vi "Begin.vi"(8 "error in":errorcluster) -> (0 "error out":errorcluster)   [LabVIEW 2015]
doc: "Called before other user functions, this VI is expected to open initial I/O refnums, load in file data, and do all program initialization. Notice that the <B>error out</B> terminal is simply used for data flow. Wiring it to other structures or subVIs ensures that this VI runs first."
uses:
  <vilib>/Rock Robotics/WPI/DriverStation/WPI_DriverStationRobotMode2.ctl
  <vilib>/Rock Robotics/WPI/CAN/TalonSRX/WPI_CANTalonSRX_APIControlMode.ctl
  <vilib>/Rock Robotics/SystemInterfaces/AI/FPGA_AIGyroChannel.ctl
  <vilib>/Rock Robotics/SystemInterfaces/DIO/FPGA_DIOChannel.ctl
  <vilib>/Rock Robotics/SystemInterfaces/DIO/FPGA_DIOPWMChannel.ctl
  <vilib>/Rock Robotics/WPI/Joystick/WPI_JoystickDeviceEnum.ctl
  <vilib>/Rock Robotics/WPI/CAN/TalonSRX/WPI_CANTalonSRX_BrakeOverride.ctl
  <vilib>/Rock Robotics/WPI/CAN/TalonSRX/WPI_CANTalonSRX_APIFeedbackSelect.ctl
  Robot Global Data.vi
  <vilib>/Rock Robotics/Network Tables/NT Write String Array.vi
  <vilib>/Rock Robotics/WPI/MotorControl/WPI_MotorControlOpenCANTalonSRX.vi
  <vilib>/Rock Robotics/WPI/Gyro/WPI_GyroAnalogOpen.vi
  <vilib>/Rock Robotics/WPI/MotorControl/WPI_MotorControlOpen VictorSP.vi
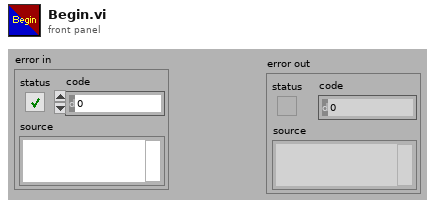
[diagram p1: front panel]
types:
  T1 = typedef "WPI_CANTalonSRX_APIFeedbackSelect.ctl" = enum16{"Digital Quadrature Encoder", "Analog Potentiometer", "Analog Encoder", "Count on Quad-A (Rising-Edge)", "Count on Quad-A (Falling-Edge)", "CTR Magnetic Enc (Absolute)", "CTR Magnetic Enc (Relative)", "Pulse Width"}
  T2 = typedef "WPI_CANTalonSRX_APIControlMode.ctl" = enum8{"Percent VBus", "Speed", "Position", "Slave", "Unchanged / Invalid", "Voltage Compensation", "Current", "Motion Profile"}
  T3 = typedef "FPGA_DIOPWMChannel.ctl" = enum8{"PWM 0", "PWM 1", "PWM 2", "PWM 3", "PWM 4", "PWM 5", "PWM 6", "PWM 7", "PWM 8", "PWM 9", "PWM MXP 0", "PWM MXP 1", "PWM MXP 2", "PWM MXP 3", "PWM MXP 4", "PWM MXP 5", "PWM MXP 6", "PWM MXP 7", "PWM MXP 8", "PWM MXP 9", "Invalid"}
  T4 = cluster{"Auton Index":i32[], "Auton Name":string[]}
  T5 = typedef "WPI_CANTalonSRX_BrakeOverride.ctl" = enum8{"No Override", "Override to Coast", "Override to Brake"}
  T6 = typedef "WPI_JoystickDeviceEnum.ctl" = enum16{"USB 0", "USB 1", "USB 2", "USB 3", "USB 4", "USB 5"}
  T7 = typedef "FPGA_DIOChannel.ctl" = enum8{"DIO 0", "DIO 1", "DIO 2", "DIO 3", "DIO 4", "DIO 5", "DIO 6", "DIO 7", "DIO 8", "DIO 9", "DIO MXP 0", "DIO MXP 1", "DIO MXP 2", "DIO MXP 3", "DIO MXP 4", "DIO MXP 5", "DIO MXP 6", "DIO MXP 7", "DIO MXP 8", "DIO MXP 9", "DIO MXP 10", "DIO MXP 11", "DIO MXP 12", "DIO MXP 13", "DIO MXP 14", "DIO MXP 15", "Invalid"}
  T8 = typedef "FPGA_AIGyroChannel.ctl" = enum8{"AI 0", "AI 1", "Invalid"}
  T9 = typedef "WPI_DriverStationRobotMode2.ctl" = enum16{"Autonomous Disabled", "Autonomous Enabled", "Teleop Disabled", "Teleop Enabled", "Disconnected", "Finish", "Test Disabled", "Test Enabled", "Emergency Stopped"}
  T10 = typedef "WPI_ServoDeviceRef.ctl" = cluster{"DeviceStatus":errorcluster, "PWM Channel":T3, "DeadBand":T11}
  T11 = typedef "WPI_PWMDeadband.ctl" = cluster{"Name":string, "maxPositivePwm":i32, "minPositivePwm":i32, "centerPwm":i32, "maxNegativePwm":i32, "minNegativePwm":i32, "angularRange":u16}
  T12 = typedef "WPI_MotorControlDeviceRef.ctl" = cluster{"DeviceStatus":errorcluster, "Type":T13, "PWM":cluster{"PWM Channel":T3, "DeadBand":T11}, "CAN":cluster{"Device Number":u8, "Control Mode":T14, "Semaphore":T15, "Max Vout":dbl, "TalonSRX Control Mode":T2}, "Invert":bool}
  T13 = typedef "WPI_MotorControlType.ctl" = enum16{"PWM", "CAN", "CANTalonSRX"}
  T14 = typedef "WPI_CANJaguar_ControlMode.ctl" = enum8{"Percent VBus", "Current", "Speed", "Position", "Voltage"}
  T15 = typedef "Semaphore RefNum" = refnum<k1>
  T16 = typedef "WPI_DigitalInputDevRef.ctl" = cluster{"DevStatus":errorcluster, "DIO Channel":T7}
  T17 = typedef "WPI_GyroDevRef.ctl" = cluster{"DevStatus":errorcluster, "Analog Channel":T18, "Offset":dbl, "Gain (VoltsPerDegree/Second)":dbl, "Gyro Type":enum16{"Analog", "XRS450"}, "Handle":i32, "SPI Bus":T19, "Device Found":bool, "Sample Rate":dbl, "Calibrate On Open":bool}
  T18 = typedef "FPGA_AIChannel.ctl" = enum8{"AI 0", "AI 1", "AI 2", "AI 3", "AI MXP 0", "AI MXP 1", "AI MXP 2", "AI MXP 3", "Invalid"}
  T19 = typedef "spi_bus.ctl" = enum16{"SPI On-Board, CS0", "SPI On-Board, CS1", "SPI On-Board, CS2", "SPI On-Board, CS3", "SPI MXP", "Invalid"}
  T20 = typedef "WPI_JoystickDevRef.ctl" = cluster{"Device":T6}
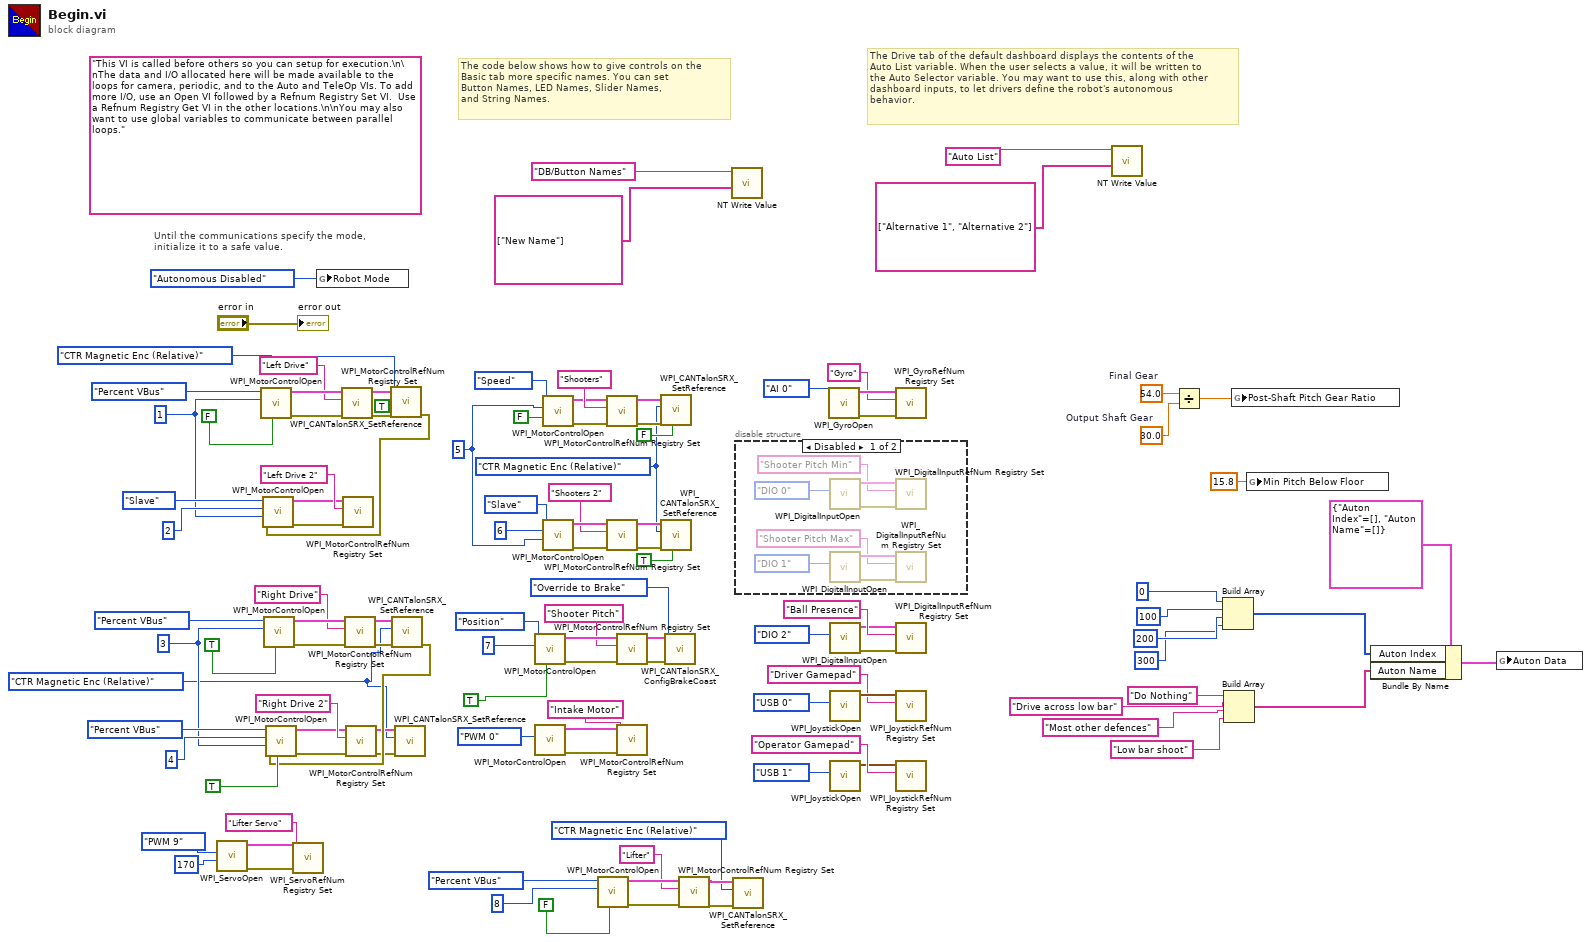
[diagram p0: block diagram]
diagram:
  w28 = WPI_CANTalonSRX_APIFeedbackSelect."CTR Magnetic Enc (Relative)" ("Feedback Reference")
  w44 = 30.0  # Output Shaft Gear
  w45 = 54.0  # Final Gear
  w54 = u8 1 ("Device Number")
  w87 = WPI_CANTalonSRX_APIFeedbackSelect."CTR Magnetic Enc (Relative)" ("Feedback Reference")
  w52 = u8 5 ("Device Number")
  w94 = u8 3 ("Device Number")
  (unwired) "This VI is called before others so you can setup for execution.\n\nThe data and I/O allocated here will be made available to the loops for camera, periodic, and to the Auto and TeleOp VIs. To add more I/O, use an Open VI followed by a Refnum Registry Set VI.  Use a Refnum Registry Get VI in the other locations.\n\nYou may also want to use global variables to communicate between parallel loops."
  # "The Drive tab of the default dashboard displays the contents of the\nAuto List variable. When the user selects a value, it will be written to\nthe Auto Selector variable. You may want to use this, along with other\ndashboard inputs, to let drivers define the robot's autonomous\nbehavior."
  # "The code below shows how to give controls on the\nBasic tab more specific names. You can set\nButton Names, LED Names, Slider Names,\nand String Names."
  # "Until the communications specify the mode,\ninitialize it to a safe value."
  n1 = call <vilib>:"WPI_ServoOpen.vi"("Angular Range"=u16 170, "PWM Channel"=FPGA_DIOPWMChannel."PWM 9") -> ("error out"=w12:errorcluster, "ServoDeviceRef"=w11:T10)  [unwired: 8 in]
  n2 = call-poly <vilib>:"WPI_MotorControlOpen.vi"("Invert"=FALSE, "Device Number"=w54, "Control Mode"=WPI_CANTalonSRX_APIControlMode."Percent VBus") -> ("error out"=w42:errorcluster, "MotorControlDeviceRef"=w60:T12)  [unwired: 7 in]
  n3 = call-poly <vilib>:"WPI_MotorControlOpen.vi"("Invert"=TRUE, "Device Number"=w94, "Control Mode"=WPI_CANTalonSRX_APIControlMode."Percent VBus") -> ("error out"=w43:errorcluster, "MotorControlDeviceRef"=w108:T12)  [unwired: 7 in]
  n4 = call <vilib>:"WPI_ServoRefNum Registry Set.vi"("error in (no error)"=w12, "refnum name"="Lifter Servo", "ServoDeviceRef"=w11) -> ()  [unwired: 7 in, 2 out]
  n5 = global write "Robot Global Data.vi" "Robot Mode"(WPI_DriverStationRobotMode2."Autonomous Disabled" ("Robot Mode")) -> ()
  n6 = call <vilib>:"WPI_MotorControlRefNum Registry Set.vi"("error in (no error)"=w42, "refnum name"="Left Drive", "MotorControlDevRef"=w60) -> ("error out"=w37:errorcluster, "MotorControlDevRef"=w38:T12)  [unwired: 7 in]
  n7 = call <vilib>:"WPI_MotorControlRefNum Registry Set.vi"("error in (no error)"=w43, "refnum name"="Right Drive", "MotorControlDevRef"=w108) -> ("error out"=w32:errorcluster, "MotorControlDevRef"=w33:T12)  [unwired: 7 in]
  n8 = call <vilib>:"WPI_CANTalonSRX_SetReference.vi"("error in (no error)"=w37, "Reverse Feedback Sensor"=TRUE, "Feedback Reference"=WPI_CANTalonSRX_APIFeedbackSelect."CTR Magnetic Enc (Relative)", "CAN Talon SRX Ref"=w38) -> ("error out"=w36:errorcluster)  [unwired: 6 in, 1 out]
  n9 = call-poly <vilib>:"WPI_MotorControlOpen.vi"("error in (no error)"=w36, "Master Device Number"=w54, "Device Number"=u8 2, "Control Mode"=WPI_CANTalonSRX_APIControlMode."Slave") -> ("error out"=w53:errorcluster, "MotorControlDeviceRef"=w57:T12)  [unwired: 6 in]
  n10 = call <vilib>:"WPI_MotorControlRefNum Registry Set.vi"("error in (no error)"=w53, "refnum name"="Left Drive 2", "MotorControlDevRef"=w57) -> ()  [unwired: 7 in, 2 out]
  n11 = call <vilib>:"WPI_CANTalonSRX_SetReference.vi"("error in (no error)"=w32, "Feedback Reference"=w28, "CAN Talon SRX Ref"=w33) -> ("error out"=w31:errorcluster)  [unwired: 7 in, 1 out]
  n12 = call-poly <vilib>:"WPI_MotorControlOpen.vi"("Invert"=TRUE, "error in (no error)"=w31, "Master Device Number"=w94, "Device Number"=u8 4, "Control Mode"=WPI_CANTalonSRX_APIControlMode."Percent VBus") -> ("error out"=w93:errorcluster, "MotorControlDeviceRef"=w105:T12)  [unwired: 5 in]
  n13 = call <vilib>:"WPI_MotorControlRefNum Registry Set.vi"("error in (no error)"=w93, "refnum name"="Right Drive 2", "MotorControlDevRef"=w105) -> ("error out"=w30:errorcluster, "MotorControlDevRef"=w29:T12)  [unwired: 7 in]
  n14 = call <vilib>:"WPI_CANTalonSRX_SetReference.vi"("error in (no error)"=w30, "Feedback Reference"=w28, "CAN Talon SRX Ref"=w29) -> ()  [unwired: 7 in, 2 out]
  n15 = call-poly <vilib>:"WPI_MotorControlOpen.vi"("Invert"=TRUE, "Device Number"=u8 7, "Control Mode"=WPI_CANTalonSRX_APIControlMode."Position") -> ("error out"=w68:errorcluster, "MotorControlDeviceRef"=w70:T12)  [unwired: 7 in]
  n16 = call-poly <vilib>:"WPI_MotorControlOpen.vi"("PWM Channel"=FPGA_DIOPWMChannel."PWM 0") -> ("error out"=w76:errorcluster, "MotorControlDeviceRef"=w75:T12)  [unwired: 9 in]
  n17 = call-poly <vilib>:"WPI_MotorControlOpen.vi"("Invert"=FALSE, "Device Number"=w52, "Control Mode"=WPI_CANTalonSRX_APIControlMode."Speed") -> ("error out"=w50:errorcluster, "MotorControlDeviceRef"=w97:T12)  [unwired: 7 in]
  n18 = call-poly <vilib>:"WPI_MotorControlOpen.vi"("Master Device Number"=w52, "Device Number"=u8 6, "Control Mode"=WPI_CANTalonSRX_APIControlMode."Slave") -> ("error out"=w51:errorcluster, "MotorControlDeviceRef"=w100:T12)  [unwired: 7 in]
  n19 = call-poly <vilib>:"WPI_MotorControlOpen.vi"("Invert"=FALSE, "Device Number"=u8 8, "Control Mode"=WPI_CANTalonSRX_APIControlMode."Percent VBus") -> ("error out"=w5:errorcluster, "MotorControlDeviceRef"=w8:T12)  [unwired: 7 in]
  n20 = call <vilib>:"WPI_MotorControlRefNum Registry Set.vi"("error in (no error)"=w50, "refnum name"="Shooters", "MotorControlDevRef"=w97) -> ("error out"=w92:errorcluster, "MotorControlDevRef"=w91:T12)  [unwired: 7 in]
  n21 = call <vilib>:"WPI_MotorControlRefNum Registry Set.vi"("error in (no error)"=w51, "refnum name"="Shooters 2", "MotorControlDevRef"=w100) -> ("error out"=w89:errorcluster, "MotorControlDevRef"=w88:T12)  [unwired: 7 in]
  n22 = call <vilib>:"WPI_MotorControlRefNum Registry Set.vi"("error in (no error)"=w68, "refnum name"="Shooter Pitch", "MotorControlDevRef"=w70) -> ("error out"=w49:errorcluster, "MotorControlDevRef"=w48:T12)  [unwired: 7 in]
  n23 = call <vilib>:"WPI_MotorControlRefNum Registry Set.vi"("error in (no error)"=w76, "refnum name"="Intake Motor", "MotorControlDevRef"=w75) -> ()  [unwired: 7 in, 2 out]
  n24 = call <vilib>:"WPI_CANTalonSRX_SetReference.vi"("Reverse Closed-Loop Output"=FALSE, "error in (no error)"=w92, "Feedback Reference"=w87, "CAN Talon SRX Ref"=w91) -> ()  [unwired: 6 in, 2 out]
  n25 = call <vilib>:"WPI_CANTalonSRX_SetReference.vi"("Reverse Closed-Loop Output"=TRUE, "error in (no error)"=w89, "Feedback Reference"=w87, "CAN Talon SRX Ref"=w88) -> ()  [unwired: 6 in, 2 out]
  n26 = call <vilib>:"WPI_CANTalonSRX_ConfigBrakeCoast.vi"("error in (no error)"=w49, "Brake / Coast Mode"=WPI_CANTalonSRX_BrakeOverride."Override to Brake", "CAN Talon SRX Ref"=w48) -> ()  [unwired: 7 in, 2 out]
  n27 = call <vilib>:"WPI_MotorControlRefNum Registry Set.vi"("error in (no error)"=w5, "refnum name"="Lifter", "MotorControlDevRef"=w8) -> ("error out"=w2:errorcluster, "MotorControlDevRef"=w3:T12)  [unwired: 7 in]
  n28 = call-poly <vilib>:"NT Write Value.vi"("String Array"=string[] ["New Name"], "Name"="DB/Button Names") -> ()  [unwired: 9 in, 1 out]
  n29 = call <vilib>:"WPI_CANTalonSRX_SetReference.vi"("error in (no error)"=w2, "Feedback Reference"=WPI_CANTalonSRX_APIFeedbackSelect."CTR Magnetic Enc (Relative)", "CAN Talon SRX Ref"=w3) -> ()  [unwired: 7 in, 2 out]
  n30 = disable-structure shown="Disabled" {
    frame Disabled {
      n31 = call <vilib>:"WPI_DigitalInputOpen.vi"("DIO Channel"=FPGA_DIOChannel."DIO 0") -> ("error out"=w123:errorcluster, "DigitalInputDevRef"=w122:T16)  [unwired: 9 in]
      n32 = call <vilib>:"WPI_DigitalInputOpen.vi"("DIO Channel"=FPGA_DIOChannel."DIO 1") -> ("error out"=w120:errorcluster, "DigitalInputDevRef"=w121:T16)  [unwired: 9 in]
      n33 = call <vilib>:"WPI_DigitalInputRefNum Registry Set.vi"("error in (no error)"=w123, "refnum name"="Shooter Pitch Min", "DigitalInputDevRef"=w122) -> ()  [unwired: 7 in, 2 out]
      n34 = call <vilib>:"WPI_DigitalInputRefNum Registry Set.vi"("error in (no error)"=w120, "refnum name"="Shooter Pitch Max", "DigitalInputDevRef"=w121) -> ()  [unwired: 7 in, 2 out]
    }
    frame Enabled {
    }
  }
  n35 = call-poly <vilib>:"WPI_GyroOpen.vi"("Analog Channel"=FPGA_AIGyroChannel."AI 0") -> ("error out"=w83:errorcluster, "GyroDevRef"=w84:T17)  [unwired: 8 in, 1 out]
  n36 = call <vilib>:"WPI_DigitalInputOpen.vi"("DIO Channel"=FPGA_DIOChannel."DIO 2") -> ("error out"=w79:errorcluster, "DigitalInputDevRef"=w78:T16)  [unwired: 9 in]
  n37 = call <vilib>:"WPI_JoystickOpen.vi"("JoystickDevice"=WPI_JoystickDeviceEnum."USB 0") -> ("JoystickDevRef"=w67:T20)  [unwired: 10 in]
  n38 = call <vilib>:"WPI_JoystickOpen.vi"("JoystickDevice"=WPI_JoystickDeviceEnum."USB 1") -> ("JoystickDevRef"=w62:T20)  [unwired: 10 in]
  n39 = call <vilib>:"WPI_GyroRefNum Registry Set.vi"("error in (no error)"=w83, "refnum name"="Gyro", "GyroDevRef"=w84) -> ()  [unwired: 7 in, 2 out]
  n40 = call <vilib>:"WPI_DigitalInputRefNum Registry Set.vi"("error in (no error)"=w79, "refnum name"="Ball Presence", "DigitalInputDevRef"=w78) -> ()  [unwired: 7 in, 2 out]
  n41 = call <vilib>:"WPI_JoystickRefNum Registry Set.vi"("refnum name"="Driver Gamepad", "JoystickDevRef"=w67) -> ()  [unwired: 8 in, 2 out]
  n42 = call <vilib>:"WPI_JoystickRefNum Registry Set.vi"("refnum name"="Operator Gamepad", "JoystickDevRef"=w62) -> ()  [unwired: 8 in, 2 out]
  n43 = call-poly <vilib>:"NT Write Value.vi"("String Array"=string[] ["Alternative 1", "Alternative 2"], "Name"="Auto List") -> ()  [unwired: 9 in, 1 out]
  n44 = Divide(x=w45, y=w44) -> (x/y=w46:dbl)
  n45 = Build Array(0, 100, 200, 300) -> (w17:i32[])
  n46 = Build Array("Do Nothing", "Drive across low bar", "Most other defences", "Low bar shoot") -> (w16:string[])
  n47 = global write "Robot Global Data.vi" "Post-Shaft Pitch Gear Ratio"(w46) -> ()
  n48 = global write "Robot Global Data.vi" "Min Pitch Below Floor"(15.8 ("Min Pitch Below Floor")) -> ()
  n49 = Bundle By Name(cluster=T4 {"Auton Index"=[], "Auton Name"=[]}, "Auton Index"=w17, "Auton Name"=w16) -> (w15:T4)
  n50 = global write "Robot Global Data.vi" "Auton Data"(w15) -> ()
  "error out" <- "error in"
